vi "computeIncrementedString.vi"(10 "Input String":string, 11 "StringIncrementAlgorithm in":refnum<class "StringIncrementAlgorithm.lvclass">) -> (2 "Incremented String":string, 3 "StringIncrementAlgorithm out":refnum<class "StringIncrementAlgorithm.lvclass">)   [LabVIEW 2014, in "UniqueName.lvlib" / "StringIncrementAlgorithm.lvclass"]
uses:
  StringIncrementAlgorithm.lvclass
  StringIncrementAlgorithm.lvclass/StringIncrementAlgorithm.ctl
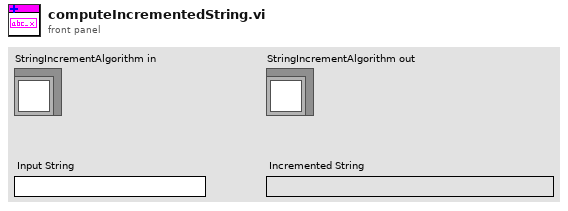
[diagram p1: front panel]
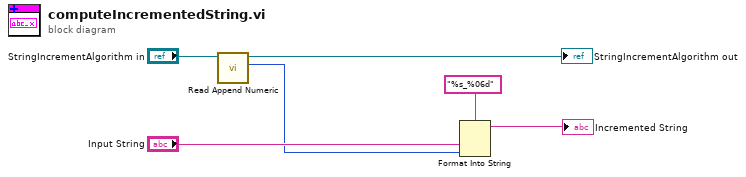
[diagram p0: block diagram]
diagram:
  n1 = call "Read Append Numeric.vi"("StringIncrementAlgorithm in"="StringIncrementAlgorithm in") -> ("Append Numeric"=w1:u32, "StringIncrementAlgorithm out"=→"StringIncrementAlgorithm out":refnum<class "StringIncrementAlgorithm.lvclass">)  [unwired: 9 in]
  n2 = Format Into String(format string="%s_%06d", "Input String", w1) -> (resulting string=→"Incremented String":string)  [unwired: 2 in, 1 out]
